vi "testRunViWithOutput.vi"(8 "error in (no error)":errorcluster) -> (0 "error out":errorcluster)   [LabVIEW 2018]
uses:
  src/SalProcess/SalProcess.lvclass
  src/VariantTool/getValFromVariant_enum.vi
  <vilib>/addons/_JKI Toolkits/Caraya/classes/Assert/Assert Equal Value_Variant.vi
  src/VariantTool/getValFromVariant_double.vi
  <vilib>/addons/_JKI Toolkits/Caraya/classes/Test/Test.lvclass
  <vilib>/addons/_JKI Toolkits/Caraya/classes/Assert/Assert.lvclass
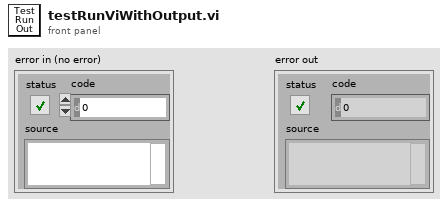
[diagram p1: front panel]
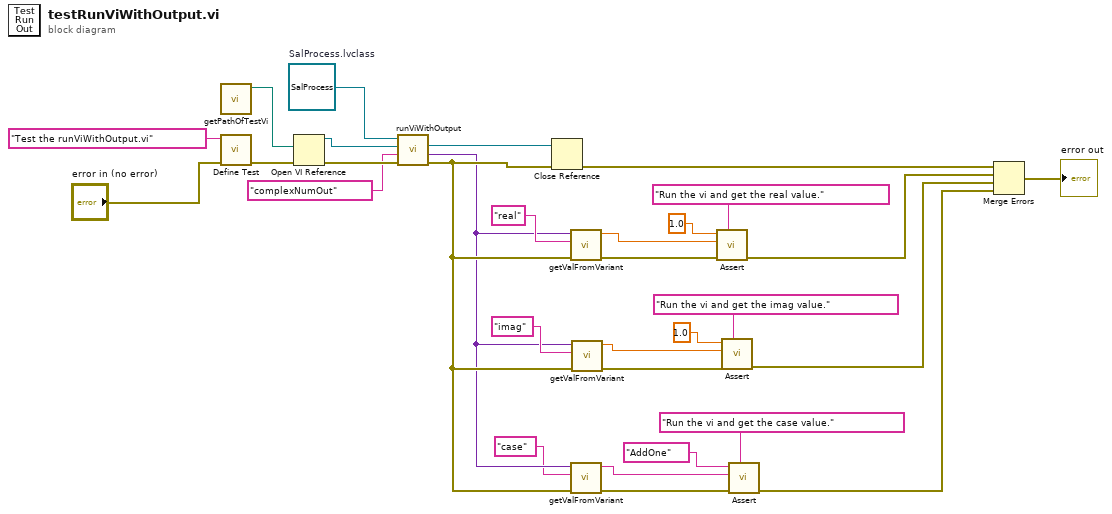
[diagram p0: block diagram]
diagram:
  w27 = refnum<class "SalProcess.lvclass"> refnum  # SalProcess.lvclass
  n1 = call "getPathOfTestVi.vi"() -> ("pathOfTestVi"=w29:path)  [unwired: 11 in]
  n2 = call <vilib>:"Define Test.vi"("error in (no error)"="error in (no error)", "Label (VI Title)"="Test the runViWithOutput.vi") -> ("error out"=w30:errorcluster)  [unwired: 9 in]
  n3 = Open VI Reference(vi path=w29, error in (no error)=w30) -> (vi reference=w26:refnum<vi>, error out=w25:errorcluster)  [unwired: 4 in]
  n4 = call "runViWithOutput.vi"("error in (no error)"=w25, "clusterNameOutput"="complexNumOut", "referenceIn"=w26, "SalProcess in"=w27) -> ("error out"=w8:errorcluster, "variant"=w7:variant, "referenceOut"=w10:refnum<vi>)  [unwired: 3 in, 2 out]
  n5 = Close Reference(reference=w10, error in (no error)=w8) -> (error out=w13:errorcluster)
  n6 = call-poly "getValFromVariant.vi"("error in (no error)"=w8, "name"="real", "variant"=w7) -> ("error out"=w21:errorcluster, "value"=w14:dbl)  [unwired: 7 in]
  n7 = call-poly "getValFromVariant.vi"("error in (no error)"=w8, "name"="case", "variant"=w7) -> ("error out"=w5:errorcluster, "value"=w4:string)  [unwired: 7 in]
  n8 = call-poly "getValFromVariant.vi"("error in (no error)"=w8, "name"="imag", "variant"=w7) -> ("error out"=w16:errorcluster, "value"=w15:dbl)  [unwired: 7 in]
  n9 = call-poly <vilib>:"Assert.vi"("Label"="Run the vi and get the real value.", "error in (no error)"=w21, "Y"=w14, "X"=1.0) -> ("error out"=w12:errorcluster)  [unwired: 7 in]
  n10 = call-poly <vilib>:"Assert.vi"("Label"="Run the vi and get the imag value.", "error in (no error)"=w16, "Y"=w15, "X"=1.0) -> ("error out"=w11:errorcluster)  [unwired: 7 in]
  n11 = call-poly <vilib>:"Assert.vi"("Label"="Run the vi and get the case value.", "error in (no error)"=w5, "Y"=w4, "X"="AddOne") -> ("error out"=w1:errorcluster)  [unwired: 7 in]
  n12 = Merge Errors(w13, w12, w11, w1) -> (→"error out":errorcluster)
